vi "CalculateExtinctionCorrectionsToDoublyChargeParticleContribution.vi"(2 "refractive index, imaginary":sgl=0.1 step=0.01 format="%.3f", 3 "refractive index, real":sgl=1.3 step=0.01 format="%.3f", 4 "Extinction ExtinctionUncertainity Size parameter and Number ofS sizes":T1={"Extinction"=[], "Extinction Uncertainty"=[], "Size parameters"=[], "Number ofSizes"=0.0, "GeometricCrossSection"=[], "Wave Length"=0.0, "SMPS Sizes"=[], "Concentration"=[], "Double Charge Correction"=FALSE, "Extincation Factor"=1.0, "Diameter Factor"=1.0, "Diameter Offset"=0.0, "Extinction Factor Flag"=FALSE, "Diameter Factor Flag"=FALSE, "Diameter Offset Flag"=FALSE, "Sizes"=[], "ExtinctionOrAbsorptionOrScattering"=0} {"ExtinctionOrAbsorptionOrScattering" scale=0.0..2.0}) -> (0 "Expected Extinction graph":cluster{"Size parameters":dbl[], dbl[]}, 1 "Expected Extinction Cross Section":sgl[](array[numeric]))   [LabVIEW 2011]
uses:
  BaesDataTypeDefinition.ctl
  <vilib>/imath/engines/lvmath2/RunTimeEngine/ErrorHandling/NIMS_Finalize Error.vi
  <vilib>/imath/engines/lvmath2/RunTimeEngine/Managers/WorkSpace/UID Generator.vi
  <vilib>/imath/engines/lvmath2/RunTimeEngine/Managers/SymbolTable/Clear UID.vi
  <vilib>/imath/engines/lvmath2/RunTimeEngine/NodeEndStatement/NIMS_NodeEndStatement_Output.vi
  <instcachedir>/0/NIMS_NodeEndStatement_Output_53EC0D466D134D7ABD903AC30B43404B.lvgen/NIMS_NodeEndStatement_Output_53EC0D466D134D7ABD903AC30B43404B_005.vi
  <vilib>/imath/engines/lvmath2/RunTimeEngine/RunTimeType/NIMS_RunTimeType_From StrictType (excl LVString).vi
  <instcachedir>/0/NIMS_RunTimeType_From StrictType (excl LVString)_46AE8B54A11948F0BCCEB8091EE7AA4C.lvgen/NIMS_RunTimeType_From StrictType (excl LVString)_46AE8B54A11948F0BCCEB8091EE7AA4C_000.vi
  <vilib>/imath/engines/lvmath2/RunTimeEngine/LocalVariableDefStatement/MC_LocalVariableDefStatement_Display.vi
  <vilib>/Analysis/baseanly.llb/Real Dot Product.vi
  <instcachedir>/0/NIMS_NodeEndStatement_Output_53EC0D466D134D7ABD903AC30B43404B.lvgen/NIMS_NodeEndStatement_Output_53EC0D466D134D7ABD903AC30B43404B_001.vi
  mie2.dll
  <vilib>/Analysis/NI_AALBase.lvlib
  <vilib>/imath/engines/lvmath2/RunTimeEngine/Managers/SymbolTable/NIMS_WorkSpace.lvlib
panel:
  out "totalscatter 3":sgl=3.7788873
  out "backscatter 3":sgl=8.098428
  out "<cos(theta)> 4":sgl=0.19839454
  out "extinction 3":sgl=1.6240653
  in  "angles (will compute\n2*angles-1 points from\n0...180 degrees)":u32=2
  out "totalscatter 2":sgl=3.7788873
  out "backscatter 2":sgl=8.098428
  out "<cos(theta)> 3":sgl=0.19839454
  out "extinction 2":sgl=1.6240653
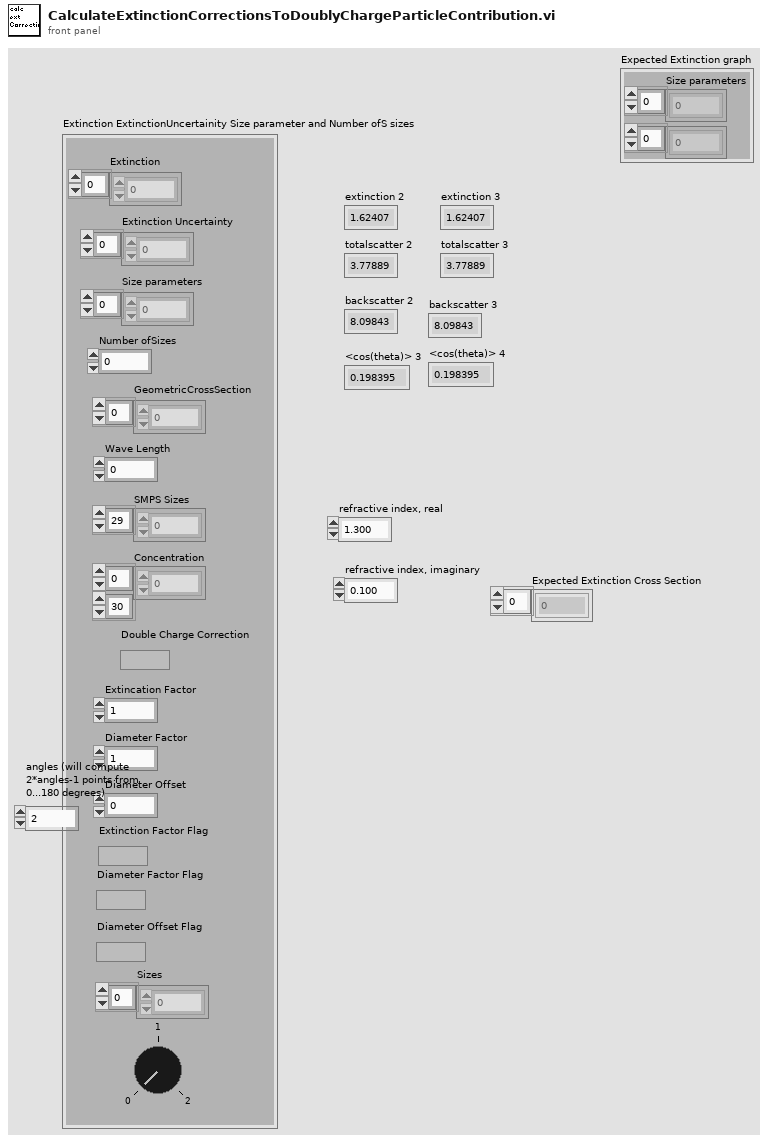
[diagram p1: front panel]
types:
  T1 = typedef "BaesDataTypeDefinition.ctl" = cluster{"Extinction":dbl[], "Extinction Uncertainty":dbl[], "Size parameters":dbl[], "Number ofSizes":dbl, "GeometricCrossSection":dbl[], "Wave Length":dbl, "SMPS Sizes":dbl[], "Concentration":dbl[][], "Double Charge Correction":bool, "Extincation Factor":dbl, "Diameter Factor":dbl, "Diameter Offset":dbl, "Extinction Factor Flag":bool, "Diameter Factor Flag":bool, "Diameter Offset Flag":bool, "Sizes":dbl[], "ExtinctionOrAbsorptionOrScattering":i8}
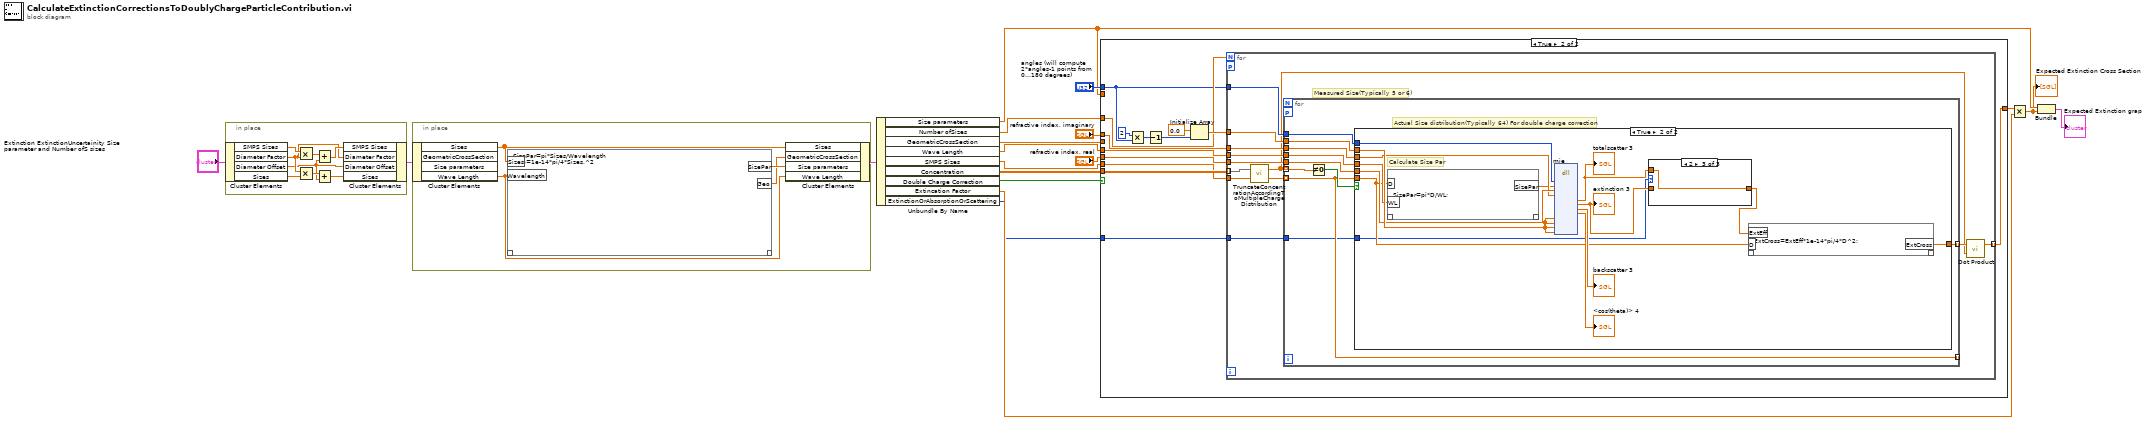
[diagram p0: block diagram]
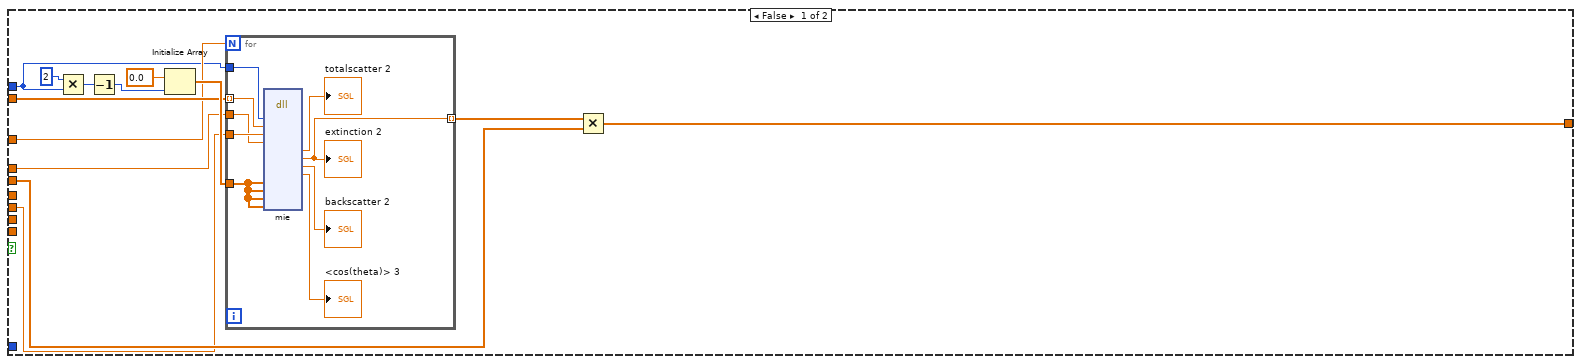
[diagram p2: hidden frame]
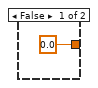
[diagram p3: hidden frame]
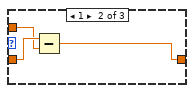
[diagram p5: hidden frame]
diagram:
  n1 = in-place {
    n2 = in-place-cluster #1("Extinction ExtinctionUncertainity Size parameter and Number ofS sizes") -> ("SMPS Sizes"=w26:dbl[], "Diameter Factor"=w22:dbl, "Diameter Offset"=w20:dbl, "Sizes"=w23:dbl[])
    n3 = Multiply(x=w26, y=w22) -> (x*y=w25:dbl[])
    n4 = Multiply(x=w22, y=w23) -> (x*y=w21:dbl[])
    n5 = Add(x=w25, y=w20) -> (x+y=w24:dbl[])
    n6 = Add(x=w21, y=w20) -> (x+y=w19:dbl[])
    n7 = in-place-cluster #1("SMPS Sizes"=w24, "Diameter Factor"=w22, "Diameter Offset"=w20, "Sizes"=w19) -> (w7:T1)
  }
  n8 = in-place {
    n9 = in-place-cluster #2(w7) -> ("Sizes"=w30:dbl[], "Wave Length"=w28:dbl)  [unwired: 2 out]
    n10 = mathscript code="SizePar=pi*Sizes/Wavelength\nGeo=1e-14*pi/4*Sizes.^2"("Sizes"=w30, "Wavelength"=w28) -> ("SizePar"=w29:dbl[], "Geo"=w27:dbl[])  [unwired: 1 in, 1 out]
    n11 = in-place-cluster #2("Sizes"=w30, "GeometricCrossSection"=w27, "Size parameters"=w29, "Wave Length"=w28) -> (w6:T1)
  }
  n12 = Unbundle By Name(w6) -> ("Size parameters"=w11:dbl[], "Number ofSizes"=w18:dbl, "GeometricCrossSection"=w17:dbl[], "Wave Length"=w12:dbl, "SMPS Sizes"=w8:dbl[], "Concentration"=w9:dbl[][], "Double Charge Correction"=w16:bool, "Extincation Factor"=w3:dbl, "ExtinctionOrAbsorptionOrScattering"=w1:i8)
  n13 = case shown="True" w16 {
    tunnel: w11 -> [w96 _]
    tunnel: w18 -> [w95 w119]
    tunnel: w17 -> [w93 _]
    tunnel: "angles (will compute\n2*angles-1 points from\n0...180 degrees)" -> [w92 w118]
    tunnel: "refractive index, imaginary" -> [w91 w117]
    tunnel: "refractive index, real" -> [w90 w116]
    tunnel: w8 -> [_ w112]
    tunnel: w12 -> [_ w115]
    tunnel: w9 -> [_ w113]
    tunnel: [w89 w114] -> w4
    tunnel: w1 -> [_ w111]
    frame False {
      n14 = Multiply(x=u32 2, y=w92) -> (x*y=w100:u32)
      n15 = Decrement(x=w100) -> (x-1=w98:u32)
      n16 = Initialize Array(sgl 0.0, w98) -> (w97:sgl[])
      n17 = for {
        N: w95 -> [_]
        tunnel: w97 -> [w108]
        tunnel: w92 -> [w107]
        tunnel: w90 -> [w106]
        tunnel: w91 -> [w105]
        tunnel: w96 -> [w104] mode=indexing
        tunnel: [w102] -> w94 mode=indexing
        n18 = dll-call lib="Z:/Downloads/Lior Segev Code Projects/RiRetrievalForLabview/mie2.dll" fn="mie"("angles"=w107, "x"=w104, "r"=w106, "i"=w105, "spol_real"=w108, "spol_imaginary"=w108, "ppol_real"=w108, "ppol_imaginary"=w108) -> ("totalscatter"=→"totalscatter 2":sgl, "extinction"=w102:sgl, "backscatter"=→"backscatter 2":sgl, "<cos(theta)>"=→"<cos(theta)> 3":sgl)  [unwired: 16 in, 2 out]
        "extinction 2" <- w102
      }
      n19 = Multiply(x=w94, y=w93) -> (x*y=w89:dbl[])
    }
    frame True {
      n20 = Multiply(x=u32 2, y=w118) -> (x*y=w123:u32)
      n21 = Decrement(x=w123) -> (x-1=w121:u32)
      n22 = Initialize Array(sgl 0.0, w121) -> (w120:sgl[])
      n23 = for {
        N: w119 -> [_]
        tunnel: w120 -> [w136]
        tunnel: w118 -> [w135]
        tunnel: w116 -> [w134]
        tunnel: w117 -> [w133]
        tunnel: w112 -> [w129]
        tunnel: w115 -> [w132]
        tunnel: w113 -> [w127] mode=indexing
        tunnel: [w131] -> w114 mode=indexing
        workers-P: _ -> [_]
        tunnel: w111 -> [w125]
        # "Measured Size(Typically 5 or 6)"
        n24 = call "TruncateConcentrationAccordingToMultipleChargeDistribution.vi"("Sizes"=w129, "Concentration"=w127) -> ("Truncated Sizes"=w128:dbl[], "Truncated Concentration"=w126:dbl[])
        n25 = for {
          tunnel: w136 -> [w146]
          tunnel: w135 -> [w145]
          tunnel: w134 -> [w144]
          tunnel: w133 -> [w143]
          tunnel: w128 -> [w138] mode=indexing
          tunnel: w132 -> [w141]
          tunnel: w126 -> [w140] mode=indexing
          tunnel: [w139] -> w130 mode=indexing
          tunnel: [w138] -> _ mode=indexing
          workers-P: _ -> [_]
          tunnel: w125 -> [w137]
          # "Actual Size distribution(Typically 64) For double charge correction"
          n26 = Not Equal To 0?(x=w140) -> (x != 0?=w142:bool)
          n27 = case shown="True" w142 {
            tunnel: w146 -> [_ w159]
            tunnel: w145 -> [_ w158]
            tunnel: w144 -> [_ w157]
            tunnel: w143 -> [_ w156]
            tunnel: w138 -> [_ w154]
            tunnel: w141 -> [_ w155]
            tunnel: [0.0 ("ExtCross") w153] -> w139
            tunnel: w137 -> [_ w148]
            frame False {
            }
            frame True {
              # "Calculate Size Par"
              n28 = mathscript code="SizePar=pi*D/WL;"("D"=w154, "WL"=w155) -> ("SizePar"=w152:dbl)  [unwired: 1 in, 1 out]
              n29 = dll-call lib="Z:/Downloads/Lior Segev Code Projects/RiRetrievalForLabview/mie2.dll" fn="mie"("angles"=w158, "x"=w152, "r"=w157, "i"=w156, "spol_real"=w159, "spol_imaginary"=w159, "ppol_real"=w159, "ppol_imaginary"=w159) -> ("totalscatter"=w149:sgl, "extinction"=w151:sgl, "backscatter"=→"backscatter 3":sgl, "<cos(theta)>"=→"<cos(theta)> 4":sgl)  [unwired: 16 in, 2 out]
              "totalscatter 3" <- w149
              "extinction 3" <- w151
              n30 = case shown="2" w148 {
                tunnel: w151 -> [w162 w165 _]
                tunnel: [w162 w163 w166] -> w150
                tunnel: w149 -> [_ w164 w166]
                frame 0, Default {
                }
                frame 1 {
                  n31 = Subtract(x=w165, y=w164) -> (x-y=w163:sgl)
                }
                frame 2 {
                }
              }
              n32 = mathscript code="ExtCross=ExtEff*1e-14*pi/4*D^2;"("ExtEff"=w150, "D"=w154) -> ("ExtCross"=w153:dbl)  [unwired: 1 in, 1 out]
            }
          }
        }
        n33 = call-poly <vilib>:"Dot Product.vi"("Y Vector"=w126, "X Vector"=w130) -> ("X * Y"=w131:dbl)  [unwired: 1 out]
      }
    }
  }
  n34 = Multiply(x=w4, y=w3) -> (x*y=w2:dbl[])
  "Expected Extinction Cross Section" <- w2
  n35 = Bundle("Size parameters"=w11, w2) -> (→"Expected Extinction graph":cluster{"Size parameters":dbl[], dbl[]})  [unwired: 1 in]
